vi "POO 1.vi"() -> ()   [LabVIEW 2020]
uses:
  Controller/Ctrl_ID.ctl
  Controller/Ctrl_States.ctl
panel:
  in  "Local":cluster{"States":T1, "ID":T2}
  out "error out":errorcluster
  in  "error in":errorcluster
  in  "Btn_Reset":bool
  in  "Btn_Read":bool
  out "Read ID":T2
  in  "Btn_write":bool
  in  "Write ID":T2
  # "Write"
  # "Read"
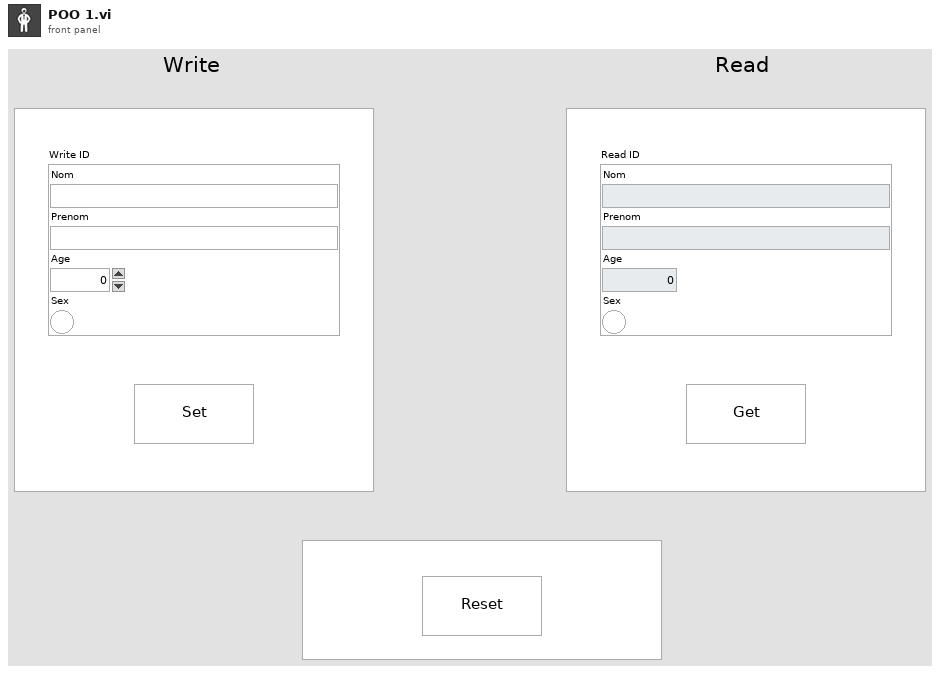
[diagram p1: front panel]
types:
  T1 = typedef "Ctrl_States.ctl" = enum16{"Idle", "Read", "Write", "Reset", "Quit"}
  T2 = typedef "Ctrl_ID.ctl" = cluster{"Nom":string, "Prenom":string, "Age":u8, "Sex":bool}
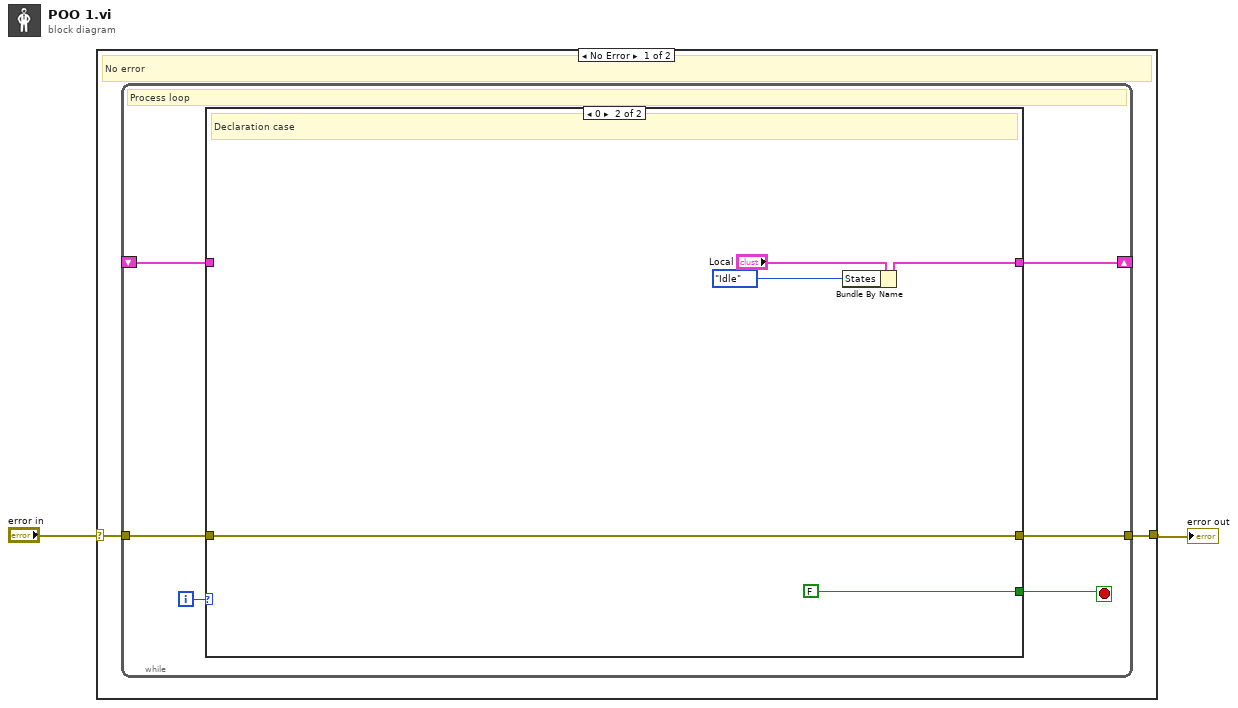
[diagram p0: block diagram]
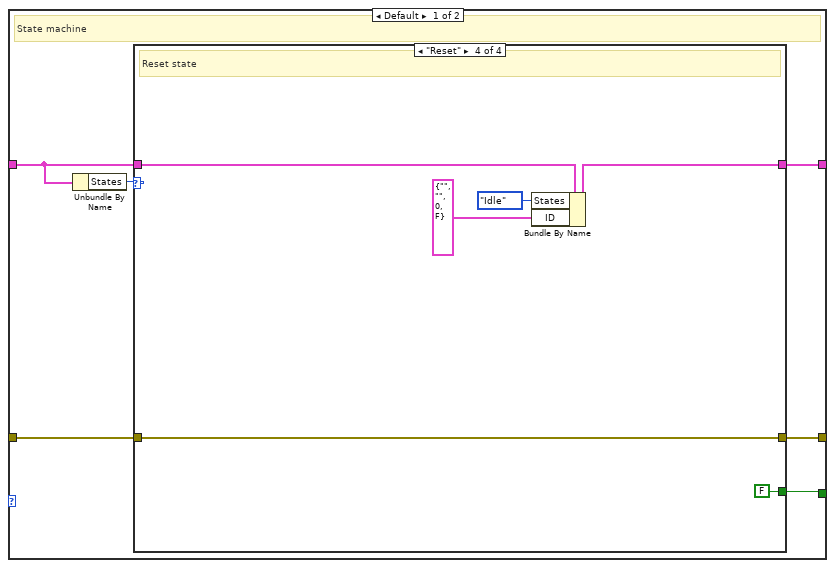
[diagram p2: hidden frame]
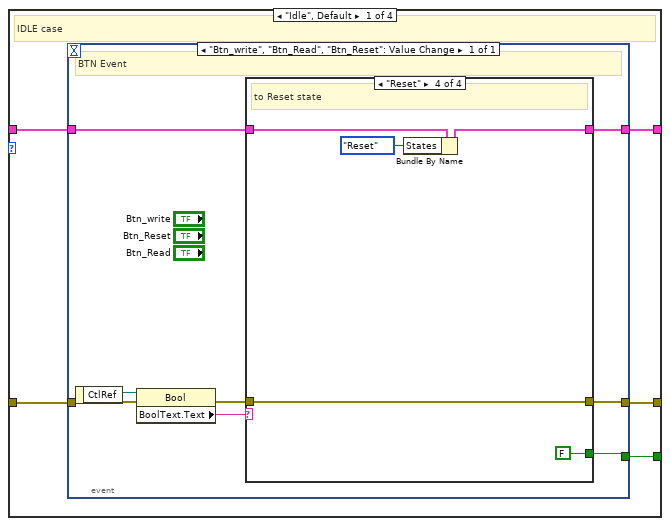
[diagram p3: hidden frame]
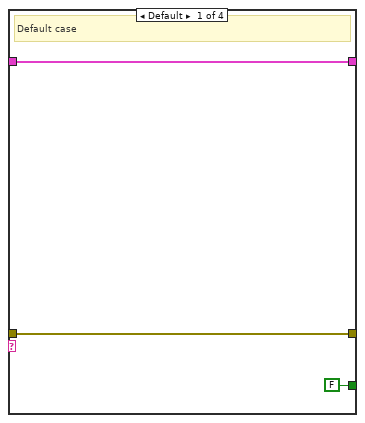
[diagram p4: hidden frame]
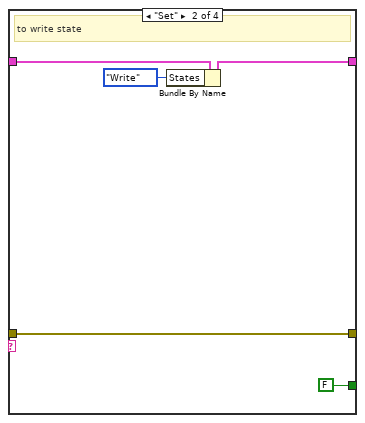
[diagram p5: hidden frame]
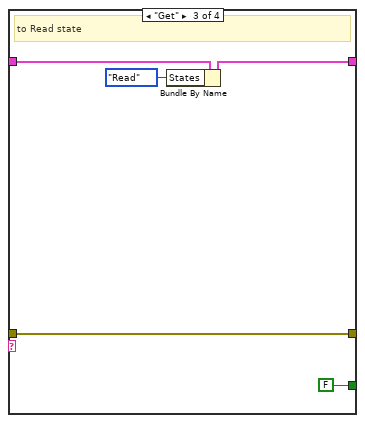
[diagram p6: hidden frame]
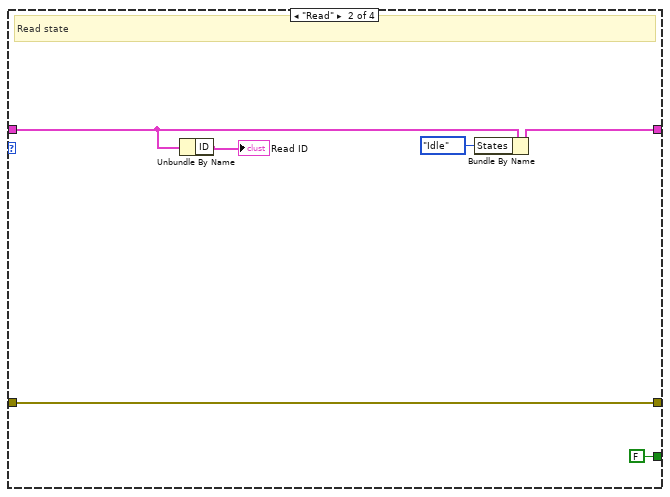
[diagram p7: hidden frame]
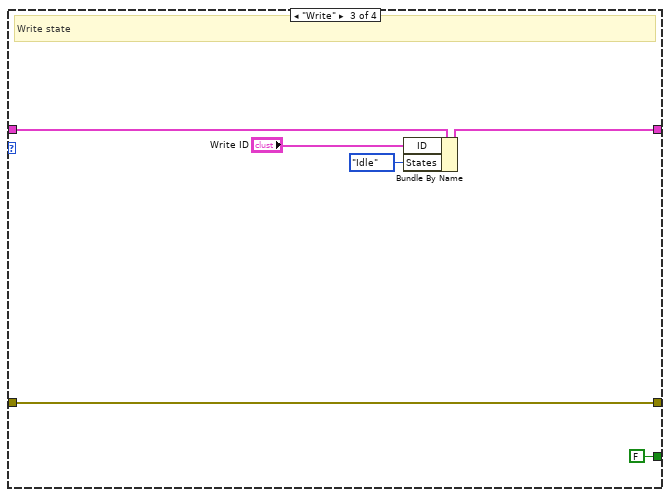
[diagram p8: hidden frame]
diagram:
  n1 = case shown="No Error" "error in" {
    selector: "error in" -> [w4 w71]
    tunnel: [w3 w71] -> w1
    frame No Error {
      # "No error"
      n2 = while {
        tunnel: w4 -> [w6]
        shift-right: [w8] -> _
        shift-left: _ -> [w7]
        tunnel: [w5] -> w3
        i -> [w10]
        stop <- w9 stop-if-true
        # "Process loop"
        n3 = case shown="0" w10 {
          tunnel: [w11 FALSE] -> w9
          tunnel: [w16 w68] -> w8
          tunnel: w7 -> [w15 _]
          tunnel: w6 -> [w13 w66]
          tunnel: [w12 w66] -> w5
          frame Default {
            # "State machine"
            n4 = Unbundle By Name(w15) -> ("States"=w14:T1)
            n5 = case shown="\"Reset\"" w14 {
              tunnel: w15 -> [w20 w51 w57 w63]
              tunnel: [w19 w49 w56 w62] -> w16
              tunnel: w13 -> [w18 w53 w59 w65]
              tunnel: [w17 w53 w59 w65] -> w12
              tunnel: [w21 FALSE FALSE FALSE] -> w11
              frame "Idle", Default {
                # "IDLE case"
                n6 = event shown="[0] \"Btn_write\", \"Btn_Read\", \"Btn_Reset\": Value Change" {
                  selector: _ -> [_]
                  dyn-events: _ -> [_]
                  timeout: _ -> [_]
                  tunnel: [w22] -> w21
                  tunnel: w20 -> [w27]
                  tunnel: [w26] -> w19
                  tunnel: w18 -> [w28]
                  tunnel: [w23] -> w17
                  event "Btn_write", "Btn_Read", "Btn_Reset": Value Change {
                    # "BTN Event"
                    n7 = event-data() -> ("CtlRef"=w29:refnum<vi>)  [unwired: 1 in]
                    n8 = property class="Bool"(reference=w29, error in=w28) -> (error out=w24:errorcluster, "BoolText.Text"=w25:string)  [unwired: 1 out]
                    n9 = case shown="\"Reset\"" w25 {
                      tunnel: w27 -> [w32 w37 w42 w47]
                      tunnel: [w32 w35 w40 w45] -> w26
                      tunnel: w24 -> [w31 w36 w41 w46]
                      tunnel: [w31 w36 w41 w46] -> w23
                      tunnel: [FALSE FALSE FALSE FALSE] -> w22
                      frame Default {
                        # "Default case"
                      }
                      frame "Set" {
                        # "to write state"
                        n10 = Bundle By Name(cluster=w37, "States"=Ctrl_States."Write") -> (w35:cluster{"States":T1, "ID":T2})
                      }
                      frame "Get" {
                        # "to Read state"
                        n11 = Bundle By Name(cluster=w42, "States"=Ctrl_States."Read") -> (w40:cluster{"States":T1, "ID":T2})
                      }
                      frame "Reset" {
                        # "to Reset state"
                        n12 = Bundle By Name(cluster=w47, "States"=Ctrl_States."Reset") -> (w45:cluster{"States":T1, "ID":T2})
                      }
                    }
                  }
                }
              }
              frame "Read" {
                # "Read state"
                n13 = Unbundle By Name(w51) -> ("ID"=→"Read ID":T2)
                n14 = Bundle By Name(cluster=w51, "States"=Ctrl_States."Idle") -> (w49:cluster{"States":T1, "ID":T2})
              }
              frame "Write" {
                # "Write state"
                n15 = Bundle By Name(cluster=w57, "ID"="Write ID", "States"=Ctrl_States."Idle") -> (w56:cluster{"States":T1, "ID":T2})
              }
              frame "Reset" {
                # "Reset state"
                n16 = Bundle By Name(cluster=w63, "States"=Ctrl_States."Idle", "ID"=T2 {"Nom"="", "Prenom"="", "Age"=0, "Sex"=FALSE}) -> (w62:cluster{"States":T1, "ID":T2})
              }
            }
          }
          frame 0 {
            # "Declaration case"
            n17 = Bundle By Name(cluster="Local", "States"=Ctrl_States."Idle") -> (w68:cluster{"States":T1, "ID":T2})
          }
        }
      }
    }
    frame Error {
    }
  }
  "error out" <- w1
